vi "Export.vi"(8 "error in":errorcluster, 11 "Objects in":T1) -> (0 "error out":errorcluster)   [LabVIEW 2015, in "tag select module editor node.lvclass"]
uses:
  tag select module editor node.lvclass
  <vilib>/NI/DCAF/Tag Editor Core/Table API/Table Manager/object ref.ctl
  <vilib>/NI/DCAF/Tag Editor Core/Configuration Editor/Classes/Engine Parent/Engine Parent Editor Node.lvclass
  <vilib>/NI/DCAF/Tag Editor Core/Configuration Editor/Classes/Module editor node/module editor node.lvclass
  <vilib>/NI/DCAF/Tag Editor Core/Table API/Table Manager/Table Manager.lvclass
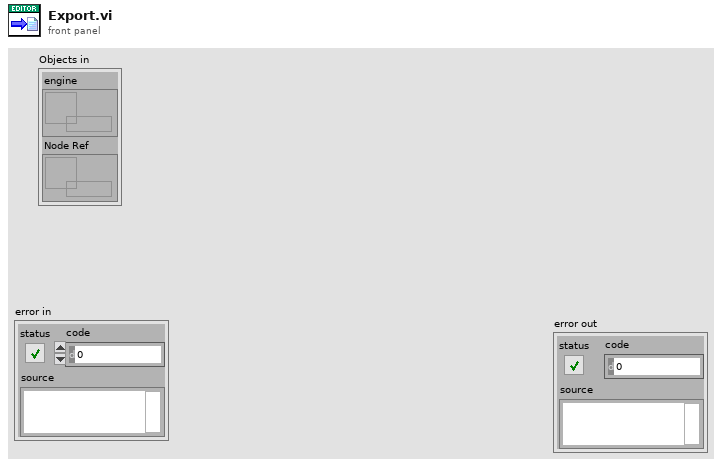
[diagram p1: front panel]
types:
  T1 = typedef "Table Manager.lvlib/Table Manager.lvclass/object ref.ctl" = cluster{"engine":refnum<data-value>, "Node Ref":refnum<data-value>}
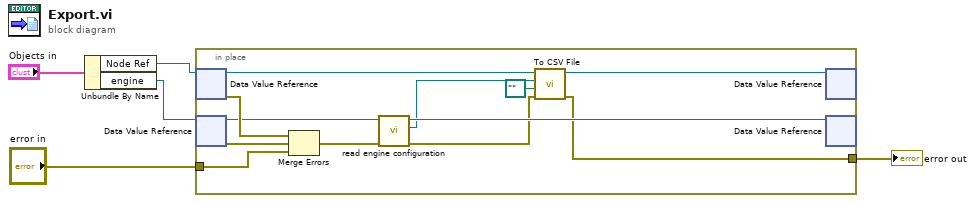
[diagram p0: block diagram]
diagram:
  n1 = Unbundle By Name("Objects in") -> ("Node Ref"=w4:refnum<data-value>, "engine"=w3:refnum<data-value>)
  n2 = in-place {
    in-place-border: "error in" -> [w15]
    in-place-border: [w7] -> w1
    n3 = in-place-dvr #1(w4) -> (w11:refnum<class "module editor node.lvclass">, w17:errorcluster)
    n4 = in-place-dvr #2(w3) -> (w13:refnum<class "Engine Parent Editor Node.lvclass">, w16:errorcluster)
    n5 = Merge Errors(w17, w16, w15) -> (w14:errorcluster)
    n6 = call <vilib>:"read engine configuration.vi"("error in"=w14, "Engine Parent Editor Node in"=w13) -> ("error out"=w9:errorcluster, "engine configuration"=w8:refnum<class "engine configuration.lvclass">, "Engine Parent Editor Node out"=w12:refnum<class "Engine Parent Editor Node.lvclass">)  [unwired: 7 in]
    n7 = call-dynamic "To CSV File.vi"("error in (no error)"=w9, "Path"=path "", "engine configuration"=w8, "module editor node in"=w11) -> ("error out"=w7:errorcluster, "module editor node out"=w10:refnum<class "module editor node.lvclass">)  [unwired: 6 in]
    n8 = in-place-dvr #1(w10) -> ()  [unwired: 2 out]
    n9 = in-place-dvr #2(w12) -> ()  [unwired: 2 out]
  }
  "error out" <- w1
